vi "Update_Current_Value_server.vi"(1 "Mode":T2(ring), 2 "Client HD name":string="G3_3 HD", 3 "Update array in":T1[](array[typedef]) {"New Value" format="%.2f"}) -> (0 "Update array out":T1[](array[typedef]) {"New Value" format="%.2f"})   [LabVIEW 2020]
uses:
  ADAM Client/Sub VIs/ADAM Controls/Update_scan_value.ctl
  ADAM_Global.vi
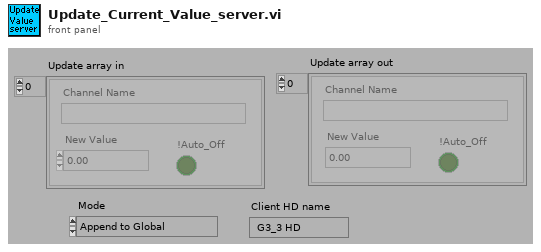
[diagram p1: front panel]
types:
  T1 = typedef "Update_scan_value.ctl" = cluster{"Channel Name":string, "New Value":dbl, "!Auto_Off":bool}
  T2 = enum16{"Append to Global", "Read Global then Clear"}
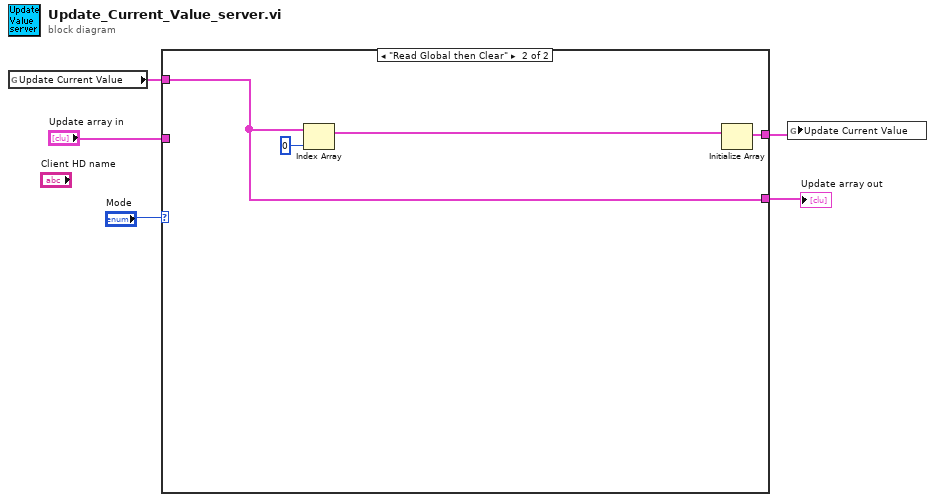
[diagram p0: block diagram]
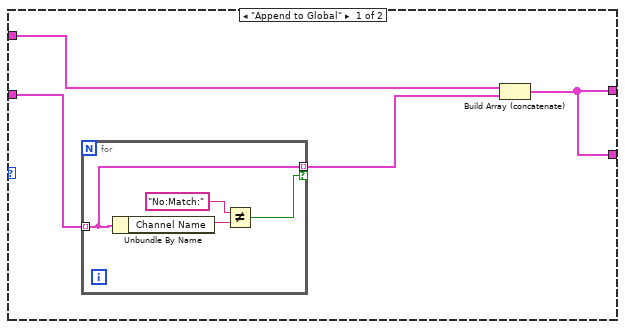
[diagram p2: hidden frame]
diagram:
  n1 = global read "ADAM_Global.vi" "Update Current Value"() -> (w5:T1[])
  n2 = case shown="\"Read Global then Clear\"" "Mode" {
    tunnel: w5 -> [w9 w14]
    tunnel: "Update array in" -> [w7 _]
    tunnel: [w8 w17] -> w2
    tunnel: [w8 w14] -> w1
    frame "Append to Global" {
      n3 = for {
        tunnel: w7 -> [w11] mode=indexing
        tunnel: [w11] -> w6 mode=indexing if=w10
        n4 = Unbundle By Name(w11) -> ("Channel Name"=w13:string)
        n5 = Not Equal?(x="No:Match:", y=w13) -> (x != y?=w10:bool)
      }
      n6 = Build Array (concatenate)(w9, w6) -> (w8:T1[])
    }
    frame "Read Global then Clear" {
      n7 = Index Array(array=w14, index=0) -> (element=w15:T1)
      n8 = Initialize Array(w15) -> (w17:T1[])  [unwired: 1 out]
    }
  }
  "Update array out" <- w1
  n9 = global write "ADAM_Global.vi" "Update Current Value"(w2) -> ()
